vi "Read Server LNA.vi"(8 "error in (no error)":errorcluster, 11 "Server Controller in":refnum<class "Server Controller.lvclass">) -> (0 "error out":errorcluster, 2 "Actor Framework:Message Enqueuer":refnum<class "Message Enqueuer.lvclass">, 3 "Server Controller out":refnum<class "Server Controller.lvclass">)   [LabVIEW 2016, in "Server Controller.lvlib" / "Server Controller.lvclass"]
uses:
  Server Controller.lvclass
  <vilib>/ActorFramework/Message Enqueuer/Message Enqueuer.lvclass
  Server Controller.lvclass/Server Controller.ctl
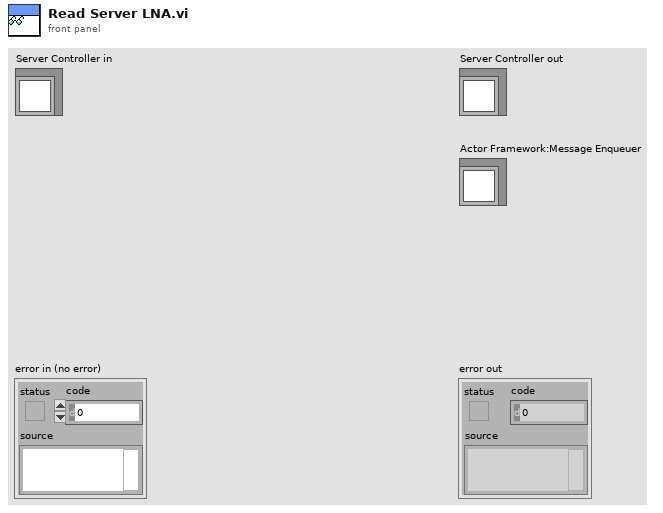
[diagram p1: front panel]
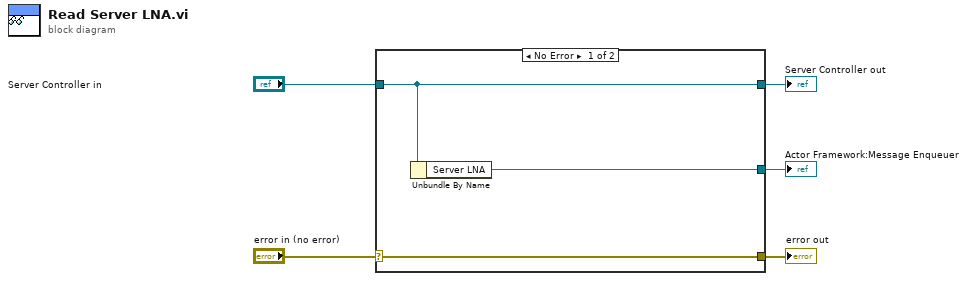
[diagram p0: block diagram]
diagram:
  n1 = case shown="No Error" "error in (no error)" {
    selector: "error in (no error)" -> [w8 w9]
    tunnel: [w8 w9] -> w4
    tunnel: [w7 w10] -> w2
    tunnel: "Server Controller in" -> [w7 w10]
    tunnel: [w6 _] -> w1
    frame No Error {
      n2 = Unbundle By Name(w7) -> ("Server LNA"=w6:refnum<class "Message Enqueuer.lvclass">)
    }
    frame Error {
    }
  }
  "error out" <- w4
  "Server Controller out" <- w2
  "Actor Framework:Message Enqueuer" <- w1
